vi "Self-Initialize Stimulator.vi"(4 "error in (no error)":errorcluster, 7 "Stimulator in":T1={"Log File In"=refnum, "Stimulator In"="", "Stimulator Mode"="", "Log Data"=FALSE, "Doublet/Triplet  Interval"=0.0, "Stim Frequency"=0.0, "N-Factor"=0, "Active Channels"=[], "Low-Frequency Channels"=[], "Stimulator State"=enum."Closed", "Mode Array"=[], "Current Array"=[], "Pulse Duration Array"=[], "VISA Timeout"=50}) -> (0 "error out":errorcluster, 1 "Write to Log":string, 2 "Response":u8, 3 "Stimulator Out":T1={"Log File In"=refnum, "Stimulator In"="", "Stimulator Mode"="", "Log Data"=FALSE, "Doublet/Triplet  Interval"=0.0, "Stim Frequency"=0.0, "N-Factor"=0, "Active Channels"=[], "Low-Frequency Channels"=[], "Stimulator State"=enum."Closed", "Mode Array"=[], "Current Array"=[], "Pulse Duration Array"=[], "VISA Timeout"=50})   [LabVIEW 2019]
uses:
  Controls/Stimulator Cluster.ctl
  Controls/Stimulator Mode.ctl
  Version 2/Data Type Defs/Pulse Mode (array).ctl
  Controls/Stim Current Array.ctl
  Controls/Pulse Duration Array.ctl
  Version 2/Data Type Defs/Obsolete/Stimulator Init Control_obs.ctl
  Version 2/Data Type Defs/Stim Init Data.ctl
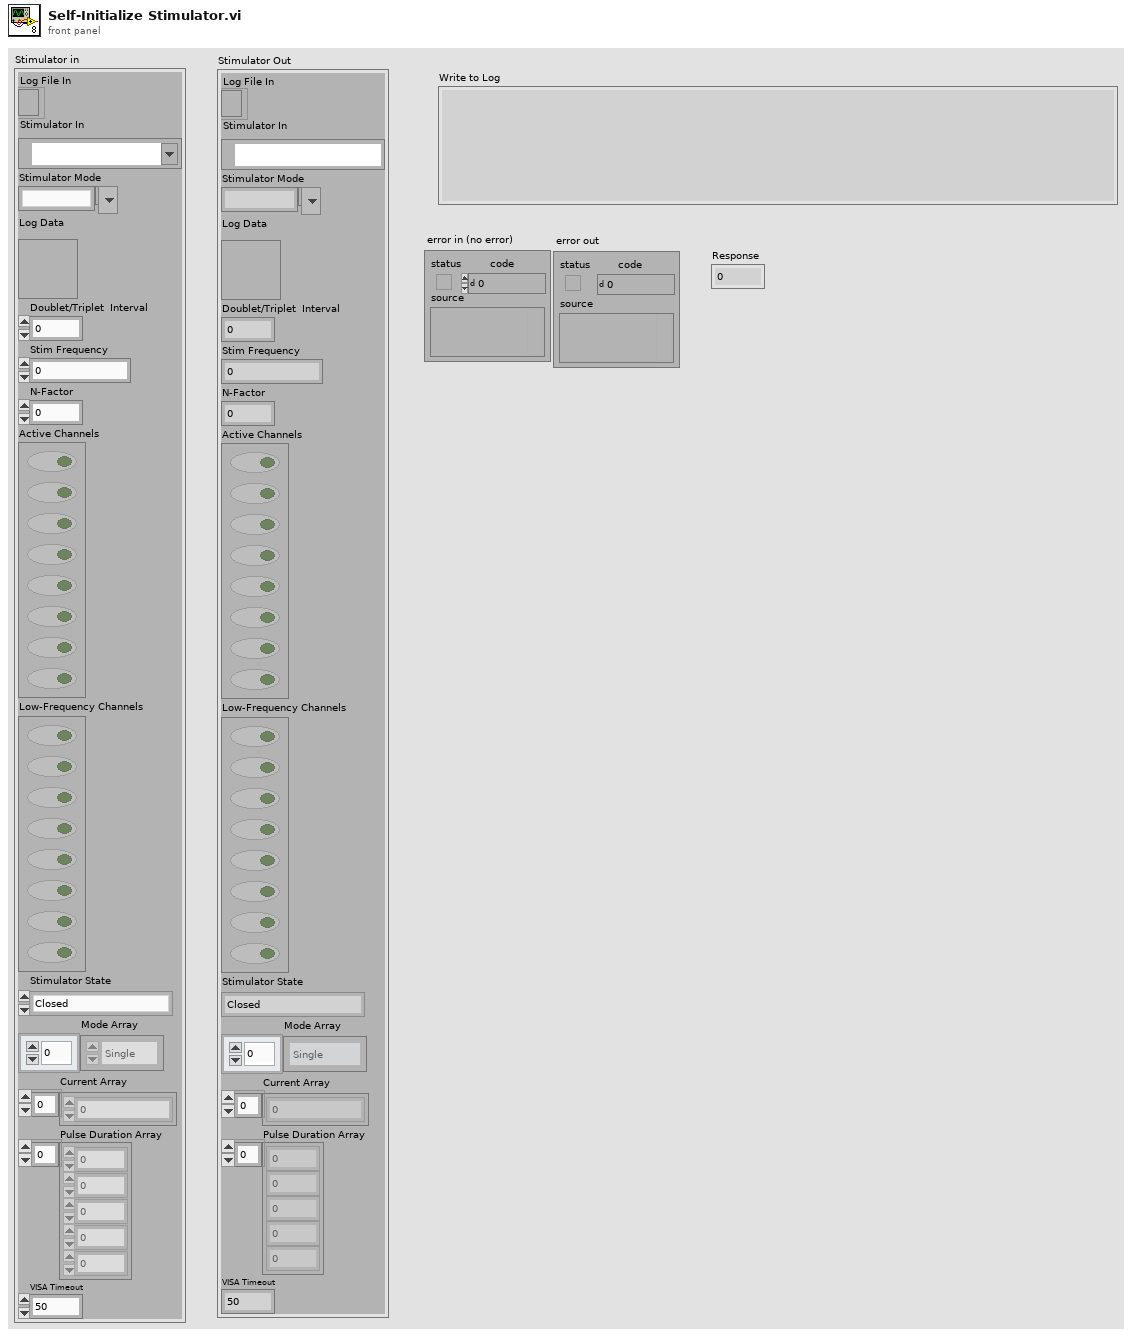
[diagram p1: front panel]
types:
  T1 = typedef "Stimulator Cluster.ctl" = cluster{"Log File In":refnum<file>, "Stimulator In":refnum<visa-resource-name>, "Stimulator Mode":T2, "Log Data":bool, "Doublet/Triplet  Interval":dbl, "Stim Frequency":dbl, "N-Factor":u8, "Active Channels":bool[], "Low-Frequency Channels":bool[], "Stimulator State":enum16{"Closed", "Open", "Initialized", "Stimulating"}, "Mode Array":T3, "Current Array":T4, "Pulse Duration Array":T5, "VISA Timeout":u32}
  T2 = typedef "Stimulator Mode.ctl" = string
  T3 = typedef "Pulse Mode (array).ctl" = enum16{"Single", "Doublet", "Triplet"}[]
  T4 = typedef "Stim Current Array.ctl" = u8[]
  T5 = typedef "Pulse Duration Array.ctl" = u32[]
  T6 = typedef "Stimulator Init Control_obs.ctl" = cluster{"Stimulator Control":cluster{"Name":refnum<visa-resource-name>, "Mode":enum16{"LIVE", "SIM"}, "Visa Timeout":u32}, "Initialization Parameters":T7}
  T7 = typedef "Stim Init Data.ctl" = cluster{"Frequency":dbl, "N Factor":u8, "D/T Int":dbl, "Active Channels":bool[], "LF Channels":bool[]}
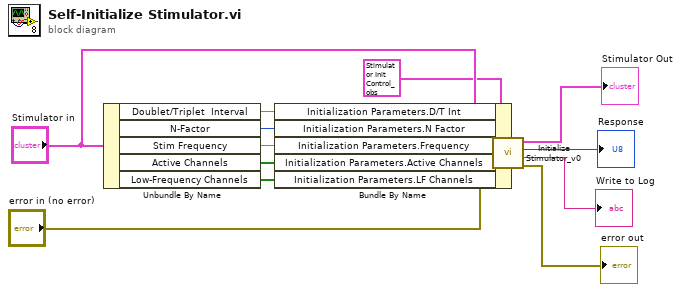
[diagram p0: block diagram]
diagram:
  n1 = Unbundle By Name("Stimulator in") -> ("Doublet/Triplet  Interval"=w10:dbl, "N-Factor"=w9:u8, "Stim Frequency"=w8:dbl, "Active Channels"=w7:bool[], "Low-Frequency Channels"=w6:bool[])
  n2 = Bundle By Name(cluster=T6 {"Stimulator Control"={"Name"="", "Mode"=enum."SIM", "Visa Timeout"=0}, "Initialization Parameters"={"Frequency"=0.0, "N Factor"=0, "D/T Int"=0.0, "Active Channels"=[TRUE, TRUE, TRUE, TRUE, TRUE], "LF Channels"=[FALSE, FALSE, FALSE, FALSE, FALSE]}} ("Initialization Parameters"), "Initialization Parameters.D/T Int"=w10, "Initialization Parameters.N Factor"=w9, "Initialization Parameters.Frequency"=w8, "Initialization Parameters.Active Channels"=w7, "Initialization Parameters.LF Channels"=w6) -> (w12:T6)
  n3 = call "Initialize Stimulator_v0.vi"("error in (no error)"="error in (no error)", "Initialization Parameters"=w12, "Stimulator"="Stimulator in") -> ("error out"=→"error out":errorcluster, "Write to Log"=→"Write to Log":string, "Response"=→"Response":u8, "Stimulator Out"=→"Stimulator Out":T1)  [unwired: 1 in]
